vi "Do.vi"(8 "error in (no error)":errorcluster, 10 "Actor in":refnum<class "Actor.lvclass">, 11 "Conceret Move In Previous Msg in":refnum<class "Conceret Move In Previous Msg.lvclass">) -> (0 "error out":errorcluster, 2 "Actor out":refnum<class "Actor.lvclass">)   [LabVIEW 2013, in "Project View.lvlib" / "Conceret Move In Previous Msg.lvclass"]
doc: "(<B>Filename</B>: Actor Framework.lvlib:Message.lvclass:Do.vi)\n\nDefines what a message does when it is received by an actor. Generally, a message instructs an actor to invoke one of its methods.\n\nBy default, this method does nothing. A child class must override it to define behavior. Create a child class by using the Actor Framework Message Maker dialog box."
uses:
  Conceret Move In Previous Msg.lvclass
  <vilib>/ActorFramework/Actor/Actor.lvclass
  Project View/Project View.lvclass
  Models/Project Model Messages/Abstract Move In Previous Msg/Abstract Move In Previous Msg.lvclass
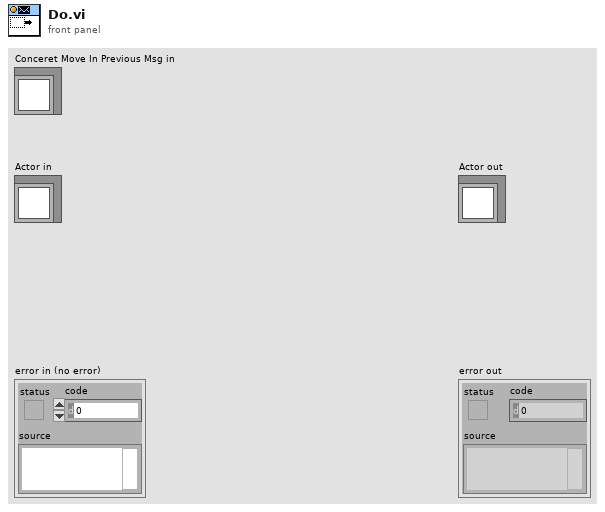
[diagram p1: front panel]
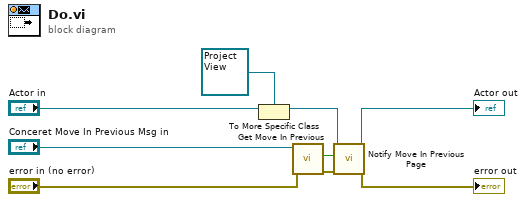
[diagram p0: block diagram]
diagram:
  n1 = To More Specific Class(target class=refnum<class "Project View.lvclass"> refnum ("Project View.lvlib:Project View.lvclass"), reference="Actor in") -> (specific class reference=w6:refnum<class "Project View.lvclass">)  [unwired: 1 in, 1 out]
  n2 = call "Get Move In Previous.vi"("error in (no error)"="error in (no error)", "Abstract Move In Previous Msg in"="Conceret Move In Previous Msg in") -> ("error out"=w5:errorcluster, "Move In Previous"=w1:bool)  [unwired: 7 in, 1 out]
  n3 = call "Notify Move In Previous Page.vi"("error in (no error)"=w5, "Move In Previous"=w1, "Project View in"=w6) -> ("error out"=→"error out":errorcluster, "Project View out"=→"Actor out":refnum<class "Project View.lvclass">)  [unwired: 7 in]
